vi "RT Audio Filter.vi"() -> ()   [LabVIEW 2016]
uses:
  <vilib>/Analysis/3filter.llb/Filter Passband Type.ctl
  <vilib>/FPGAPlugInAG/myRIO-1900/niLvFpga_Open_myRIO-1900.vi
  <vilib>/rvi/interface/common/dynamic/niFpgaDynamicAddResources.vi
  <vilib>/imath/engines/lvmath2/RunTimeEngine/BuiltInFunctions/length/NIMS_length(GV).vi
  <instcachedir>/0/NIMS_length(GV)_08A3D13377FD4E4B96F5795FBF3698FA.lvgen/NIMS_length(GV)_08A3D13377FD4E4B96F5795FBF3698FA_003.vi
  <vilib>/imath/engines/lvmath2/RunTimeEngine/RangeToken/NIMS_Range.vi
  <instcachedir>/0/NIMS_Range_A7C094595B484CA7AF10685B02D808ED.lvgen/NIMS_Range_A7C094595B484CA7AF10685B02D808ED_001.vi
  <vilib>/imathl/engines/lvmath/Functions/Error Handling/Create Error.vi
  <vilib>/imath/engines/lvmath2/RunTimeEngine/ArithmeticOperatorToken/NIMS_ArithmeticOperator_times.vi
  <instcachedir>/0/NIMS_ArithmeticOperator_times_953B34F74CAC448FB707D816A29CC5F0.lvgen/NIMS_ArithmeticOperator_times_953B34F74CAC448FB707D816A29CC5F0_009.vi
  <vilib>/imath/engines/lvmath2/RunTimeEngine/NodeEndStatement/NIMS_NodeEndStatement_Output.vi
  <instcachedir>/0/NIMS_NodeEndStatement_Output_53EC0D466D134D7ABD903AC30B43404B.lvgen/NIMS_NodeEndStatement_Output_53EC0D466D134D7ABD903AC30B43404B_005.vi
  <vilib>/imath/engines/lvmath2/RunTimeEngine/ErrorHandling/NIMS_Finalize Error.vi
  <vilib>/Utility/error.llb/Error Cluster From Error Code.vi
  <vilib>/rvi/errors/niLvFpgaAdjustHostInterfaceError.vi
  <vilib>/Analysis/3filter.llb/Butterworth Filter (DBL).vi
  <vilib>/imath/engines/lvmath2/RunTimeEngine/BuiltInFunctions/iir_butterord/NIMS_iir_butterord.vi
  <vilib>/imath/engines/lvmath2/RunTimeEngine/ErrorHandling/NIMS_Create Error From Enums.vi
  <vilib>/imath/engines/lvmath2/RunTimeEngine/BuiltInFunctions/iir_butter/NIMS_[2o]_iir_butter(I32,V).vi
  <vilib>/imath/engines/lvmath2/RunTimeEngine/ErrorHandling/NIMS_Error From Error Code.vi
  <vilib>/imath/engines/lvmath2/RunTimeEngine/BuiltInFunctions/filter/NIMS_filter(GV,GV,GV,GV,Str).vi
  <instcachedir>/0/NIMS_filter(GV,GV,GV,GV,Str)_434E59EE96884CB3BC5141C85D3A0B2F.lvgen/NIMS_filter(GV,GV,GV,GV,Str)_434E59EE96884CB3BC5141C85D3A0B2F_000.vi
  <vilib>/imath/engines/lvmath2/RunTimeEngine/BuiltInFunctions/iir_butter/NIMS_[2o]_iir_butter(I32,V,Str).vi
  <vilib>/FPGAPlugInAG/Dynamic/niLvFpga_Close_Dynamic.vi
  <vilib>/rvi/interface/nirviOpenFPGA/nirviOpenFPGA.xnode
  FPGA Bitfiles/FPGA Audio Streaming (with LEDs).lvbitx
  FPGA Audio Streaming.vi
  <vilib>/rvi/interface/nirviReadWriteControl/nirviReadWriteControl.xnode
  <vilib>/rvi/interface/nirviCloseFPGA/nirviCloseFPGA.xnode
  <vilib>/Analysis/NI_AALBase.lvlib
  <vilib>/rvi/interface/Simulation/niFpgaSimulationCallBeginRW.vi
  NiFpgaLv.dll
panel:
  in  "alpha":dbl(knob) scale=0.0..1.0
  in  "fx":dbl(knob) scale=0.0..100.0
  in  "fc [Hz]":dbl(knob)=218.02067540995574 scale=100.0..1600.0
  in  "delta f":dbl(slide)=2.9591836734693877 scale=0.0..10.0
  in  "fm [Hz]":dbl(slide)=2.4489795918367347 scale=0.0..30.0
  in  "efekt":string(combo)
  in  "Level wielokrotne [dB]":dbl(slide)=-0.5102040816326532
  in  "Time 2":u16(knob)=1 scale=0.0..6.0
  in  "Time":u16(knob)=1 scale=0.0..6.0
  in  "Level [dB]":dbl(slide)=-0.5102040816326532
  in  "Pitch":dbl(knob)=100.0 scale=0.0..1600.0
  in  "rate [Hz]":dbl(slide) scale=0.0..30.0
  in  "depth [dB]":dbl(slide) scale=0.0..10.0
  in  "stop 2":bool
  in  "Gain [dB]":dbl(slide) scale=-10.0..5.0
  in  "Mode Select":bool
  in  "Midtone":dbl(slide)=1.0 scale=0.0..1.0
  in  "Treble":dbl(slide)=1.0 scale=0.0..1.0
  in  "Bass":dbl(slide)=1.0 scale=0.0..1.0
  out "Model of Computation":string="Graphical Data Flow"
  in  "Sample Rate (Hz)":dbl=44101.0
  out "Audio Spectrum":dynamicdata(graph)=[{"t0"=timestamp(0 s since 1904-01-01), "dt"=4.991624221844934, "Y"=array[4418 elements], "attributes"=variant("NI_ChannelName"=variant(string "FFT - (RMS)"))}, {"t0"=timestamp(0 s since 1904-01-01), "dt"=4.991624221844934, "Y"=array[4418 elements], "attributes"=variant("NI_ChannelName"=variant(string "FFT - (RMS)"))}]
  in  "Read Rate (Hz)":dbl=5.0
  in  "stop":bool
  # "Audio Equilizer Control"
  # "Application Control"
  # "Tremollo"
  # "Echo"
  # "Echo wielokrotne"
  # "Signal * sin"
  # "Vibrato"
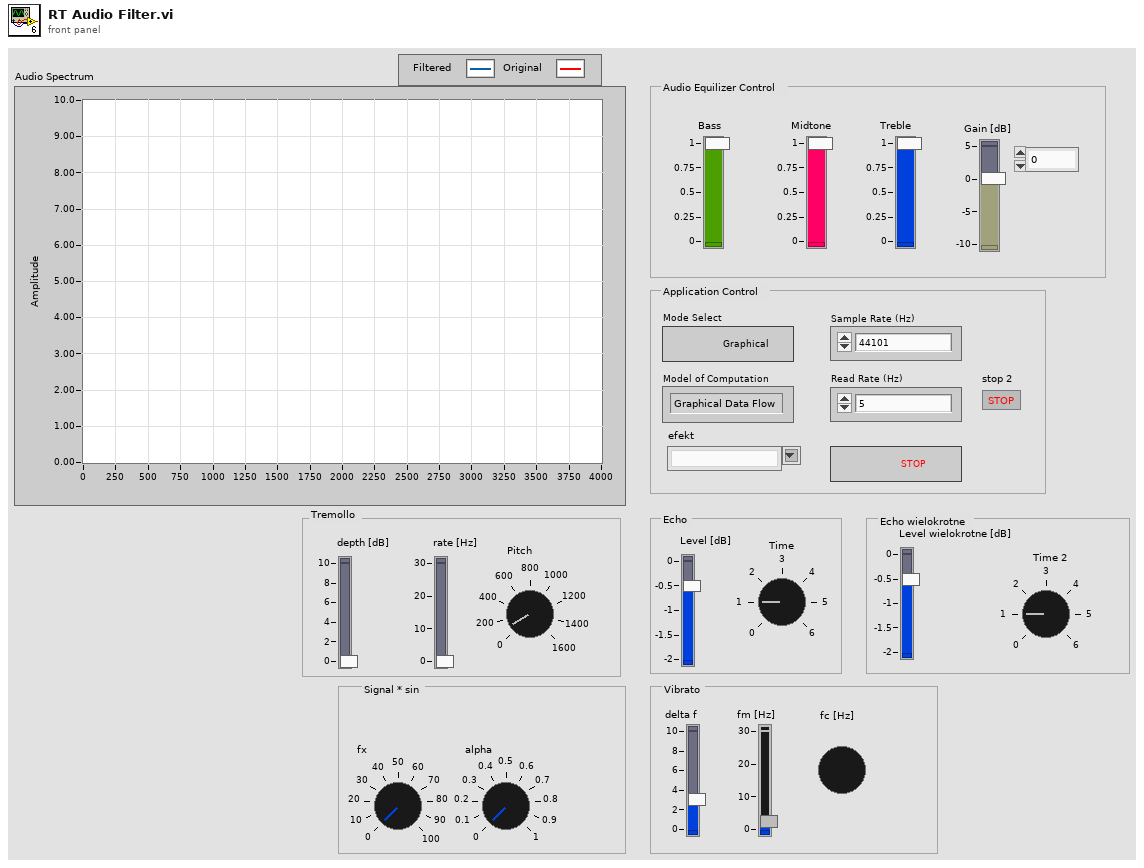
[diagram p1: front panel]
types:
  T1 = typedef "NI_AALBase.lvlib/Filter Passband Type.ctl" = enum32{"Lowpass", "Highpass", "Bandpass", "Bandstop"}
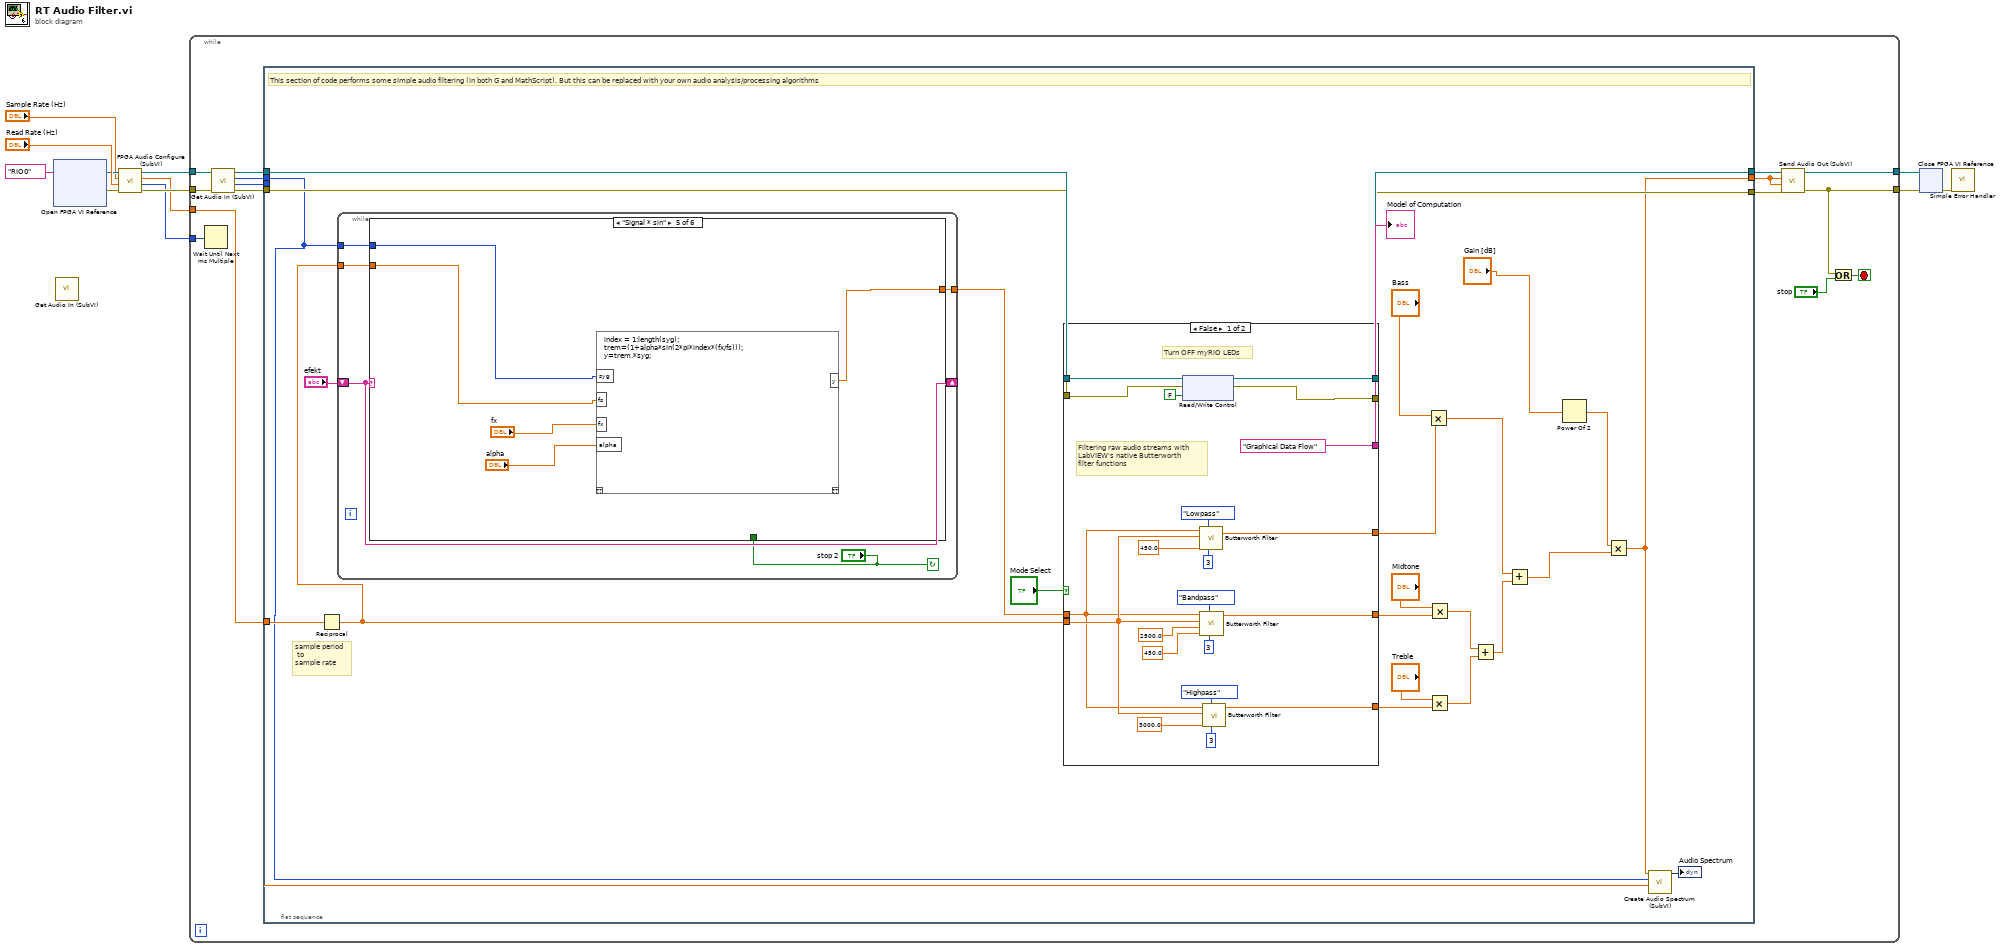
[diagram p0: block diagram]
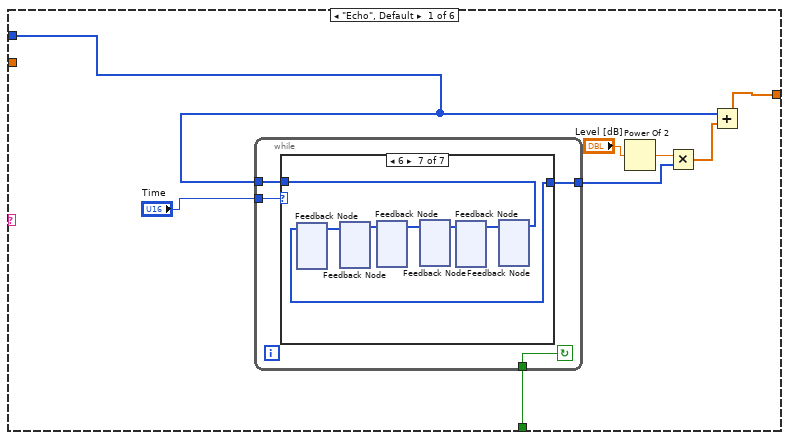
[diagram p2: hidden frame]
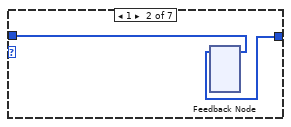
[diagram p4: hidden frame]
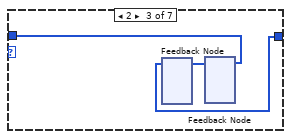
[diagram p5: hidden frame]
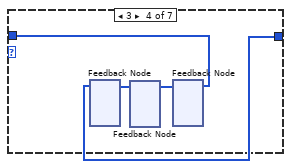
[diagram p6: hidden frame]
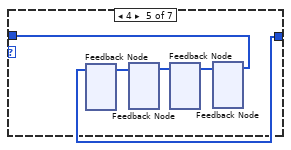
[diagram p7: hidden frame]
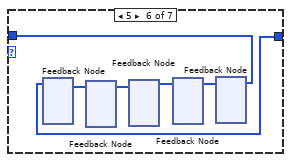
[diagram p8: hidden frame]
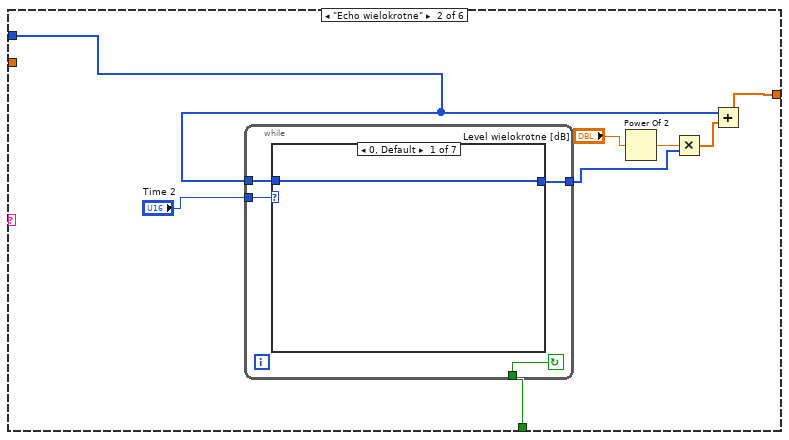
[diagram p9: hidden frame]
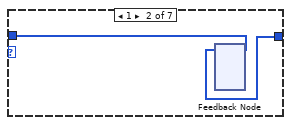
[diagram p10: hidden frame]
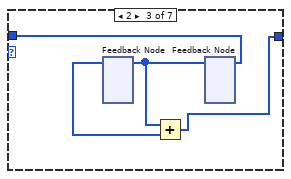
[diagram p11: hidden frame]
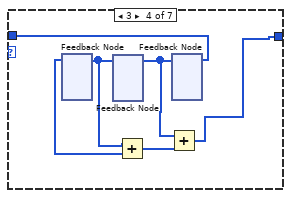
[diagram p12: hidden frame]
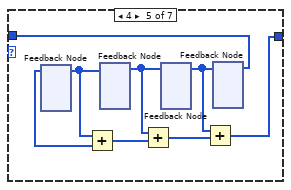
[diagram p13: hidden frame]
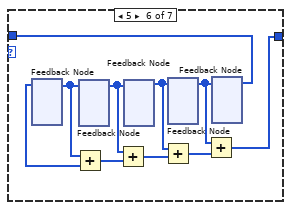
[diagram p14: hidden frame]
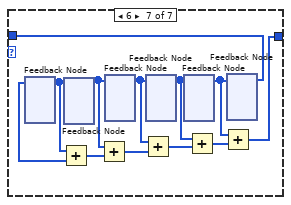
[diagram p15: hidden frame]
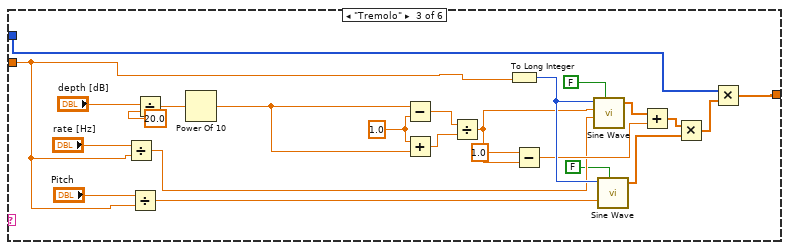
[diagram p16: hidden frame]
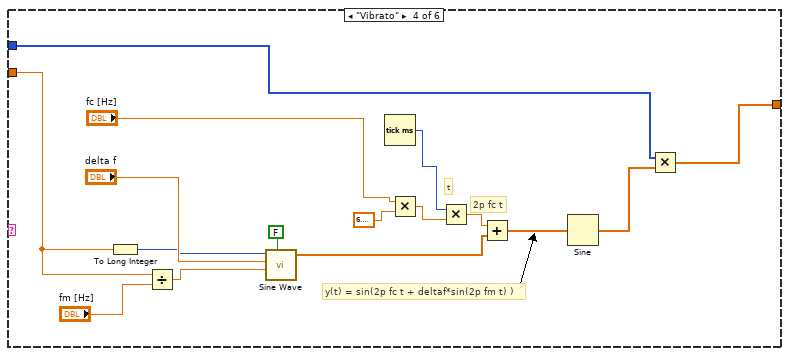
[diagram p17: hidden frame]
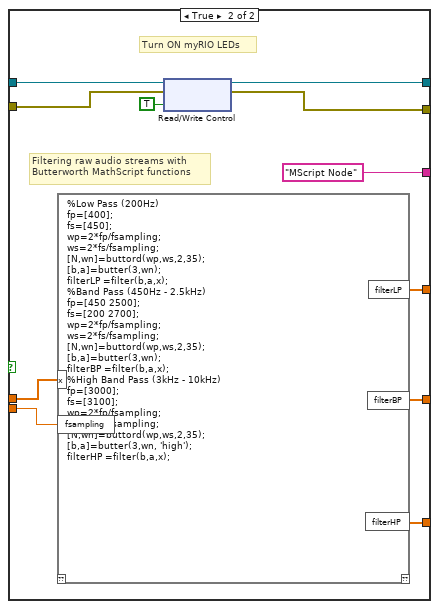
[diagram p19: hidden frame]
diagram:
  n1 = xnode "Open FPGA VI Reference"("resource name"=tag "RIO0") -> ("FPGA VI Reference Out"=w5:refnum<k20>, "error out"=w12:errorcluster)  [unwired: 1 in]
  n2 = call "Get Audio In (SubVI).vi"() -> ()  [unwired: 8 in, 4 out]
  n3 = call "FPGA Audio Configure (SubVI).vi"("error in (no error)"=w12, "Read Rate (Hz)"="Read Rate (Hz)", "Audio Sample Rate (Hz)"="Sample Rate (Hz)", "Refnum in"=w5) -> ("error out"=w7:errorcluster, "Required loop period (ms)"=w2:u32, "Audio dt (ms)"=w3:dbl, "Refnum out"=w11:refnum<k20>)  [unwired: 4 in]
  n4 = while {
    tunnel: w11 -> [w24]
    tunnel: [w22] -> w10
    tunnel: [w18] -> w9
    tunnel: w2 -> [w23]
    tunnel: w7 -> [w25]
    tunnel: w3 -> [w21]
    stop <- w26 stop-if-true
    n5 = Wait Until Next ms Multiple(millisecond multiple=w23) -> ()  [unwired: 1 out]
    n6 = call "Get Audio In (SubVI).vi"("error in (no error)"=w25, "Refnum in"=w24) -> ("error out"=w16:errorcluster, "Right Audio In"=w13:i16[], "Left Audio In"=w19:i16[], "Refnum out"=w17:refnum<k20>)  [unwired: 6 in]
    n7 = flat-sequence {
      tunnel: w21 -> [w33]
      tunnel: [w36] -> w20
      tunnel: w19 -> [w30]
      tunnel: w17 -> [w41]
      tunnel: w16 -> [w40]
      tunnel: [w39] -> w15
      tunnel: [w38] -> w14
      tunnel: w13 -> [_]
      frame #0 {
        # "sample period\n to\nsample rate"
        # "This section of code performs some simple audio filtering (in both G and MathScript). But this can be replaced with your own audio analysis/processing algorithms"
        n8 = Reciprocal(x=w33) -> (1/x=w32:dbl)
        n9 = while {
          shift-right: [w55] -> _
          shift-left: "efekt" -> [w55]
          tunnel: w30 -> [w58]
          tunnel: [w57] -> w31
          tunnel: w32 -> [w56]
          stop <- "stop 2" continue-if-true
          n10 = case shown="\"Signal * sin\"" w55 {
            tunnel: [w66 w105 w155 w179 w194 w272] -> w57
            tunnel: w58 -> [w61 w104 w176 w181 w198 w272]
            tunnel: w56 -> [_ _ w156 w183 w197 _]
            tunnel: "stop 2" -> [w59 w103 _ _ _ _]
            frame "Echo", Default {
              n11 = while {
                tunnel: "Time" -> [w70]
                tunnel: w61 -> [w69]
                tunnel: [w68] -> w60
                tunnel: w59 -> [w67]
                stop <- w67 continue-if-true
                n12 = case shown="6" w70 {
                  tunnel: w69 -> [w71 w73 w74 w79 w81 w89 w94]
                  tunnel: [w71 w72 w75 w77 w82 w86 w95] -> w68
                  frame 0, Default {
                  }
                  frame 1 {
                    n13 = feedback-in #1(w73) -> ()
                    n14 = feedback #1() -> (w72:i16[])  [unwired: 1 in]
                  }
                  frame 2 {
                    n15 = feedback #2() -> (w75:i16[])  [unwired: 1 in]
                    n16 = feedback #3() -> (w76:i16[])  [unwired: 1 in]
                    n17 = feedback-in #2(w76) -> ()
                    n18 = feedback-in #3(w74) -> ()
                  }
                  frame 3 {
                    n19 = feedback #4() -> (w77:i16[])  [unwired: 1 in]
                    n20 = feedback #5() -> (w78:i16[])  [unwired: 1 in]
                    n21 = feedback-in #4(w78) -> ()
                    n22 = feedback #6() -> (w80:i16[])  [unwired: 1 in]
                    n23 = feedback-in #5(w80) -> ()
                    n24 = feedback-in #6(w79) -> ()
                  }
                  frame 4 {
                    n25 = feedback #7() -> (w82:i16[])  [unwired: 1 in]
                    n26 = feedback #8() -> (w84:i16[])  [unwired: 1 in]
                    n27 = feedback-in #7(w84) -> ()
                    n28 = feedback #9() -> (w83:i16[])  [unwired: 1 in]
                    n29 = feedback-in #8(w83) -> ()
                    n30 = feedback #10() -> (w85:i16[])  [unwired: 1 in]
                    n31 = feedback-in #9(w85) -> ()
                    n32 = feedback-in #10(w81) -> ()
                  }
                  frame 5 {
                    n33 = feedback #11() -> (w86:i16[])  [unwired: 1 in]
                    n34 = feedback #12() -> (w87:i16[])  [unwired: 1 in]
                    n35 = feedback-in #11(w87) -> ()
                    n36 = feedback #13() -> (w90:i16[])  [unwired: 1 in]
                    n37 = feedback-in #12(w90) -> ()
                    n38 = feedback #14() -> (w88:i16[])  [unwired: 1 in]
                    n39 = feedback-in #13(w88) -> ()
                    n40 = feedback #15() -> (w91:i16[])  [unwired: 1 in]
                    n41 = feedback-in #14(w91) -> ()
                    n42 = feedback-in #15(w89) -> ()
                  }
                  frame 6 {
                    n43 = feedback #16() -> (w95:i16[])  [unwired: 1 in]
                    n44 = feedback #17() -> (w96:i16[])  [unwired: 1 in]
                    n45 = feedback-in #16(w96) -> ()
                    n46 = feedback #18() -> (w92:i16[])  [unwired: 1 in]
                    n47 = feedback-in #17(w92) -> ()
                    n48 = feedback #19() -> (w97:i16[])  [unwired: 1 in]
                    n49 = feedback-in #18(w97) -> ()
                    n50 = feedback #20() -> (w93:i16[])  [unwired: 1 in]
                    n51 = feedback-in #19(w93) -> ()
                    n52 = feedback #21() -> (w98:i16[])  [unwired: 1 in]
                    n53 = feedback-in #20(w98) -> ()
                    n54 = feedback-in #21(w94) -> ()
                  }
                }
              }
              n55 = Power Of 2(x="Level [dB]") -> (2^x=w63:dbl)
              n56 = Multiply(x=w63, y=w60) -> (x*y=w65:dbl[])
              n57 = Add(x=w61, y=w65) -> (x+y=w66:dbl[])
            }
            frame "Echo wielokrotne" {
              n58 = while {
                tunnel: "Time 2" -> [w110]
                tunnel: w104 -> [w109]
                tunnel: [w108] -> w100
                tunnel: w103 -> [w107]
                stop <- w107 continue-if-true
                n59 = case shown="0, Default" w110 {
                  tunnel: w109 -> [w111 w113 w117 w123 w131 w141 w153]
                  tunnel: [w111 w112 w114 w118 w127 w132 w149] -> w108
                  frame 0, Default {
                  }
                  frame 1 {
                    n60 = feedback-in #22(w113) -> ()
                    n61 = feedback #22() -> (w112:i16[])  [unwired: 1 in]
                  }
                  frame 2 {
                    n62 = feedback #23() -> (w116:i16[])  [unwired: 1 in]
                    n63 = feedback #24() -> (w115:i16[])  [unwired: 1 in]
                    n64 = feedback-in #23(w115) -> ()
                    n65 = Add(x=w115, y=w116) -> (x+y=w114:i16[])
                    n66 = feedback-in #24(w117) -> ()
                  }
                  frame 3 {
                    n67 = feedback #25() -> (w121:i16[])  [unwired: 1 in]
                    n68 = feedback #26() -> (w122:i16[])  [unwired: 1 in]
                    n69 = feedback-in #25(w122) -> ()
                    n70 = Add(x=w122, y=w121) -> (x+y=w120:i16[])
                    n71 = feedback #27() -> (w119:i16[])  [unwired: 1 in]
                    n72 = feedback-in #26(w119) -> ()
                    n73 = Add(x=w119, y=w120) -> (x+y=w118:i16[])
                    n74 = feedback-in #27(w123) -> ()
                  }
                  frame 4 {
                    n75 = feedback #28() -> (w124:i16[])  [unwired: 1 in]
                    n76 = feedback #29() -> (w130:i16[])  [unwired: 1 in]
                    n77 = feedback-in #28(w130) -> ()
                    n78 = Add(x=w130, y=w124) -> (x+y=w125:i16[])
                    n79 = feedback #30() -> (w129:i16[])  [unwired: 1 in]
                    n80 = feedback-in #29(w129) -> ()
                    n81 = Add(x=w129, y=w125) -> (x+y=w126:i16[])
                    n82 = feedback #31() -> (w128:i16[])  [unwired: 1 in]
                    n83 = feedback-in #30(w128) -> ()
                    n84 = Add(x=w128, y=w126) -> (x+y=w127:i16[])
                    n85 = feedback-in #31(w131) -> ()
                  }
                  frame 5 {
                    n86 = feedback #32() -> (w140:i16[])  [unwired: 1 in]
                    n87 = feedback #33() -> (w139:i16[])  [unwired: 1 in]
                    n88 = feedback-in #32(w139) -> ()
                    n89 = Add(x=w139, y=w140) -> (x+y=w137:i16[])
                    n90 = feedback #34() -> (w138:i16[])  [unwired: 1 in]
                    n91 = feedback-in #33(w138) -> ()
                    n92 = Add(x=w138, y=w137) -> (x+y=w135:i16[])
                    n93 = feedback #35() -> (w136:i16[])  [unwired: 1 in]
                    n94 = feedback-in #34(w136) -> ()
                    n95 = Add(x=w136, y=w135) -> (x+y=w133:i16[])
                    n96 = feedback #36() -> (w134:i16[])  [unwired: 1 in]
                    n97 = feedback-in #35(w134) -> ()
                    n98 = Add(x=w134, y=w133) -> (x+y=w132:i16[])
                    n99 = feedback-in #36(w141) -> ()
                  }
                  frame 6 {
                    n100 = feedback #37() -> (w147:i16[])  [unwired: 1 in]
                    n101 = feedback #38() -> (w148:i16[])  [unwired: 1 in]
                    n102 = feedback-in #37(w148) -> ()
                    n103 = Add(x=w148, y=w147) -> (x+y=w146:i16[])
                    n104 = feedback #39() -> (w145:i16[])  [unwired: 1 in]
                    n105 = feedback-in #38(w145) -> ()
                    n106 = Add(x=w145, y=w146) -> (x+y=w152:i16[])
                    n107 = feedback #40() -> (w144:i16[])  [unwired: 1 in]
                    n108 = feedback-in #39(w144) -> ()
                    n109 = Add(x=w144, y=w152) -> (x+y=w151:i16[])
                    n110 = feedback #41() -> (w143:i16[])  [unwired: 1 in]
                    n111 = feedback-in #40(w143) -> ()
                    n112 = Add(x=w143, y=w151) -> (x+y=w150:i16[])
                    n113 = feedback #42() -> (w142:i16[])  [unwired: 1 in]
                    n114 = feedback-in #41(w142) -> ()
                    n115 = Add(x=w142, y=w150) -> (x+y=w149:i16[])
                    n116 = feedback-in #42(w153) -> ()
                  }
                }
              }
              n117 = Power Of 2(x="Level wielokrotne [dB]") -> (2^x=w102:dbl)
              n118 = Multiply(x=w102, y=w100) -> (x*y=w99:dbl[])
              n119 = Add(x=w104, y=w99) -> (x+y=w105:dbl[])
            }
            frame "Tremolo" {
              w170 = 1.0 ("y")
              n120 = Divide(x="rate [Hz]", y=w156) -> (x/y=w158:dbl)
              n121 = Divide(x="Pitch", y=w156) -> (x/y=w159:dbl)
              n122 = Divide(x="depth [dB]", y=20.0) -> (x/y=w168:dbl)
              n123 = Power Of 10(x=w168) -> (10^x=w171:dbl)
              n124 = Subtract(x=w171, y=w170) -> (x-y=w172:dbl)
              n125 = Add(x=w170, y=w171) -> (x+y=w173:dbl)
              n126 = Divide(x=w172, y=w173) -> (x/y=w165:dbl)
              n127 = To Long Integer(number=w156) -> (32bit integer=w175:i32)
              n128 = Subtract(x=1.0, y=w165) -> (x-y=w164:dbl)
              n129 = call <vilib>:"Sine Wave.vi"("samples"=w175, "amplitude"=w165, "frequency"=w158, "reset phase"=FALSE) -> ("sine wave"=w163:dbl[])  [unwired: 1 in, 2 out]
              n130 = call <vilib>:"Sine Wave.vi"("samples"=w175, "frequency"=w159, "reset phase"=FALSE) -> ("sine wave"=w174:dbl[])  [unwired: 2 in, 2 out]
              n131 = Add(x=w163, y=w164) -> (x+y=w162:dbl[])
              n132 = Multiply(x=w162, y=w174) -> (x*y=w154:dbl[])
              n133 = Multiply(x=w176, y=w154) -> (x*y=w155:dbl[])
            }
            frame "Vibrato" {
              # "y(t) = sin(2p fc t + deltaf*sin(2p fm t) )"
              # "2p fc t"
              # "t"
              n134 = To Long Integer(number=w183) -> (32bit integer=w182:i32)
              n135 = Divide(x=w183, y="fm [Hz]") -> (x/y=w184:dbl)
              n136 = call <vilib>:"Sine Wave.vi"("samples"=w182, "amplitude"="delta f", "frequency"=w184, "reset phase"=FALSE) -> ("sine wave"=w188:dbl[])  [unwired: 1 in, 2 out]
              n137 = Tick Count (ms)() -> (millisecond timer value=w178:u32)
              n138 = Multiply(x="fc [Hz]", y=6.283185307179586) -> (x*y=w189:dbl)
              n139 = Multiply(x=w178, y=w189) -> (x*y=w192:dbl)
              n140 = Add(x=w192, y=w188) -> (x+y=w191:dbl[])
              n141 = Sine(x=w191) -> (sin(x)=w180:dbl[])
              n142 = Multiply(x=w181, y=w180) -> (x*y=w179:dbl[])
            }
            frame "Signal * sin" {
              n143 = mathscript code="index = 1:length(syg);\ntrem=(1+alpha*sin(2*pi*index*(fx/fs)));\ny=trem.*syg;"("syg"=w198, "fs"=w197, "fx"="fx", "alpha"="alpha") -> ("y"=w194:dbl[])  [unwired: 1 in, 1 out]
            }
            frame "No Effect" {
            }
          }
        }
        n144 = case shown="False" "Mode Select" {
          tunnel: [w293 w302] -> w46
          tunnel: [w290 w303] -> w45
          tunnel: [w273 w304] -> w44
          tunnel: ["Graphical Data Flow" ("Mode") "MScript Node" ("Mode")] -> w43
          tunnel: w32 -> [w283 w300]
          tunnel: w31 -> [w279 w299]
          tunnel: w41 -> [w278 w298]
          tunnel: w40 -> [w277 w297]
          tunnel: [w275 w295] -> w39
          tunnel: [w276 w294] -> w38
          frame False {
            # "Turn OFF myRIO LEDs"
            # "Filtering raw audio streams with \nLabVIEW's native Butterworth \nfilter functions"
            n145 = xnode "Read/Write Control"("FPGA VI Reference In"=w278, "error in"=w277, "LEDs On?"=FALSE) -> ("FPGA VI Reference Out"=w275:refnum<k20>, "error out"=w276:errorcluster)
            n146 = call-poly <vilib>:"Butterworth Filter.vi"("order"=3, "filter type"=Filter_Passband_Type."Lowpass", "low cutoff freq: fl"=450.0, "sampling freq: fs"=w283, "X"=w279) -> ("Filtered X"=w293:dbl[])  [unwired: 3 in, 1 out]
            n147 = call-poly <vilib>:"Butterworth Filter.vi"("order"=3, "filter type"=Filter_Passband_Type."Bandpass", "low cutoff freq: fl"=450.0, "high cutoff freq: fh"=2500.0, "sampling freq: fs"=w283, "X"=w279) -> ("Filtered X"=w290:dbl[])  [unwired: 2 in, 1 out]
            n148 = call-poly <vilib>:"Butterworth Filter.vi"("order"=3, "filter type"=Filter_Passband_Type."Highpass", "low cutoff freq: fl"=3000.0 ("high cutoff freq: fh"), "sampling freq: fs"=w283, "X"=w279) -> ("Filtered X"=w273:dbl[])  [unwired: 3 in, 1 out]
          }
          frame True {
            # "Turn ON myRIO LEDs"
            # "Filtering raw audio streams with \nButterworth MathScript functions"
            n149 = mathscript code="%Low Pass (200Hz)\nfp=[400]; \nfs=[450]; \nwp=2*fp/fsampling; \nws=2*fs/fsampling; \n[N,wn]=buttord(wp,ws,2,35);\n[b,a]=butter(3,wn);\nfilterLP =filter(b,a,x);\n%Band Pass (450Hz - 2.5kHz)\nfp=[450 2500]; \nfs=[200 2700]; \nwp=2*fp/fsampling; \nws=2*fs/fsampling; \n[N,wn]=buttord(wp,ws,2,35);\n[b,a]=butter(3,wn);\nfilterBP =filter(b,a,x);\n%High Band Pass (3kHz - 10kHz)\nfp=[3000]; \nfs=[3100]; \nwp=2*fp/fsampling; \nws=2*fs/fsampling; \n[N,wn]=buttord(wp,ws,2,35);\n[b,a]=butter(3,wn, 'high');\nfilterHP =filter(b,a,x);"("x"=w299, "fsampling"=w300) -> ("filterLP"=w302:dbl[], "filterBP"=w303:dbl[], "filterHP"=w304:dbl[])  [unwired: 1 in, 1 out]
            n150 = xnode "Read/Write Control"("FPGA VI Reference In"=w298, "error in"=w297, "LEDs On?"=TRUE) -> ("FPGA VI Reference Out"=w295:refnum<k20>, "error out"=w294:errorcluster)
          }
        }
        "Model of Computation" <- w43
        n151 = Multiply(x="Bass", y=w46) -> (x*y=w47:dbl[])
        n152 = Multiply(x="Treble", y=w44) -> (x*y=w49:dbl[])
        n153 = Multiply(x="Midtone", y=w45) -> (x*y=w50:dbl[])
        n154 = Add(x=w50, y=w49) -> (x+y=w48:dbl[])
        n155 = Add(x=w47, y=w48) -> (x+y=w37:dbl[])
        n156 = Power Of 2(x="Gain [dB]") -> (2^x=w35:dbl)
        n157 = Multiply(x=w35, y=w37) -> (x*y=w36:dbl[])
        n158 = call "Create Audio Spectrum (SubVI).vi"("Sample Period (ms)"=w33, "Raw Audio"=w30, "Filtered Audio"=w36) -> ("FFT Out"=→"Audio Spectrum":dynamicdata)  [unwired: 8 in]
      }
    }
    n159 = call "Send Audio Out (SubVI).vi"("error in (no error)"=w14, "Right Audio Out"=w20, "Left Audio Out"=w20, "Refnum in"=w15) -> ("error out"=w18:errorcluster, "Refnum out"=w22:refnum<k20>)  [unwired: 6 in]
    n160 = Or(x=w18, y="stop") -> (x .or. y?=w26:bool)
  }
  n161 = xnode "Close FPGA VI Reference"("FPGA VI Reference In"=w10, "error in"=w9) -> ("error out"=w1:errorcluster)
  n162 = call <vilib>:"Simple Error Handler.vi"("error in (no error)"=w1) -> ()  [unwired: 4 in, 5 out]
